vi "Update Cluster.vi"(7 "Element to Update":enum16{"<None>", "Name", "Age", "Is Married?"}(ring)=enum."Age", 8 "Is Married?":bool, 9 "Age":u8=23, 10 "Name":string="Adam", 11 "Customer Data in":T1={"Name"="Adam", "Age"=0, "Is Married?"=TRUE, "Number of Updates"=7}) -> (3 "Customer Data out":T1={"Name"="Adam", "Age"=23, "Is Married?"=TRUE, "Number of Updates"=8})   [LabVIEW 2019]
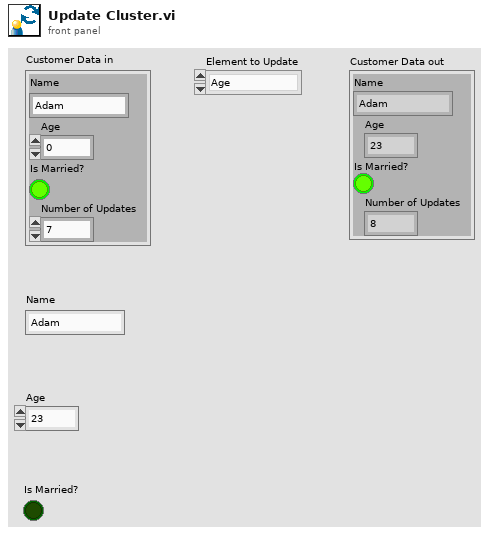
[diagram p1: front panel]
types:
  T1 = cluster{"Name":string, "Age":u8, "Is Married?":bool, "Number of Updates":i32}
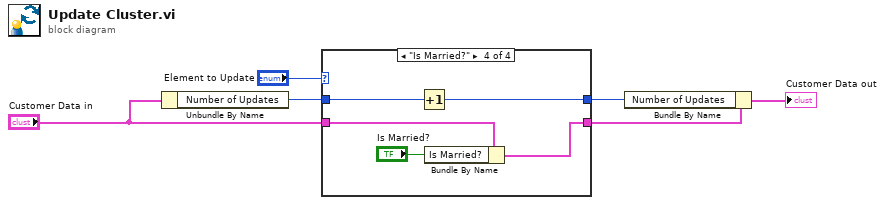
[diagram p0: block diagram]
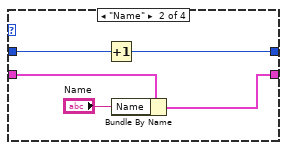
[diagram p3: hidden frame]
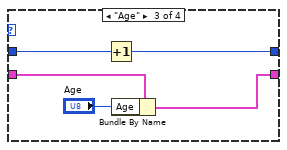
[diagram p4: hidden frame]
diagram:
  n1 = Unbundle By Name("Customer Data in") -> ("Number of Updates"=w3:i32)
  n2 = case shown="\"Is Married?\"" "Element to Update" {
    tunnel: "Customer Data in" -> [w8 w13 w18 w23]
    tunnel: [w8 w11 w17 w22] -> w5
    tunnel: w3 -> [w7 w10 w15 w20]
    tunnel: [w7 w9 w14 w19] -> w2
    frame "<None>", Default {
    }
    frame "Name" {
      n3 = Increment(x=w10) -> (x+1=w9:i32)
      n4 = Bundle By Name(cluster=w13, "Name"="Name") -> (w11:T1)
    }
    frame "Age" {
      n5 = Increment(x=w15) -> (x+1=w14:i32)
      n6 = Bundle By Name(cluster=w18, "Age"="Age") -> (w17:T1)
    }
    frame "Is Married?" {
      n7 = Increment(x=w20) -> (x+1=w19:i32)
      n8 = Bundle By Name(cluster=w23, "Is Married?"="Is Married?") -> (w22:T1)
    }
  }
  n9 = Bundle By Name(cluster=w5, "Number of Updates"=w2) -> (→"Customer Data out":T1)
